vi "ir_laser_test.vi"() -> ()   [LabVIEW 2009]
uses:
  <vilib>/Utility/file.llb/Read From Spreadsheet File (string).vi
  <vilib>/Utility/error.llb/DialogType.ctl
  <vilib>/DAQmx/read.llb/DAQmx Read (Analog 2D DBL NChan NSamp).vi
  <vilib>/DAQmx/write.llb/DAQmx Write (Analog 1D DBL 1Chan NSamp).vi
  <vilib>/DAQmx/configure/timing.llb/DAQmx Timing (Sample Clock).vi
  <vilib>/DAQmx/create/channels.llb/DAQmx Create Channel (AO-Voltage-Basic).vi
  <vilib>/DAQmx/create/channels.llb/DAQmx Create Channel (AI-Voltage-Basic).vi
  <vilib>/Utility/file.llb/Write To Spreadsheet File (DBL).vi
  <vilib>/Analysis/NI_AALBase.lvlib
panel:
  in  "Start":bool
  in  "Exit":bool
  out "Selected pulse duration":dbl
  in  "Enable temp jump":bool
  in  "Select temperature jump":string(combo)
  in  "Cell name":string
  out "File overwritten":bool
  in  "Calculate Ea":bool
  out "standard error":string
  out "standard output":string
  in  "Activation energy":dbl=77000.0 caption="Activation energy [J/mol]" min=1000.0 max=2000000.0
  out "Estimated temperature":dbl[](graph)
  out "Laser control generated":dbl[](graph)
  in  "time between short pulses":dbl=1.0 caption="Time between short pulses [s]" format="%0.2p"
  in  "short pulse duration":dbl=1.0 caption="Short pulse duration [s]" format="%0.2p"
  in  "n short pulses":i32=3
  in  "Signal":u16(ring)=1 items=["Pulse train", "Simple pulse"]
  out "Current laser power [W]":dbl
  in  "Laser power [W]":dbl[](array[numeric]) min=0.0 max=10.0
  in  "repetitions":i32=3
  in  "Save file":bool=TRUE
  in  "filename":path
  out "Laser [W]":dbl[](graph) caption="Laser control"
  out "Temperature":dbl[](graph)
  out "Current [pA]":dbl[](graph) caption="Current"
  in  "Recording  duration":dbl=10.0 caption="Duration [s]" min=4.1 max=60.0 format="%0.2p"
  in  "Pulse duration":dbl=1.0 caption="Pulse duration [s]" min=0.001 max=1.5 format="%0.2p"
  in  "Amplitude":dbl=1.0 caption="Amplitude [W]" format="%0.2p"
  out "Measurement":dbl[][](graph)
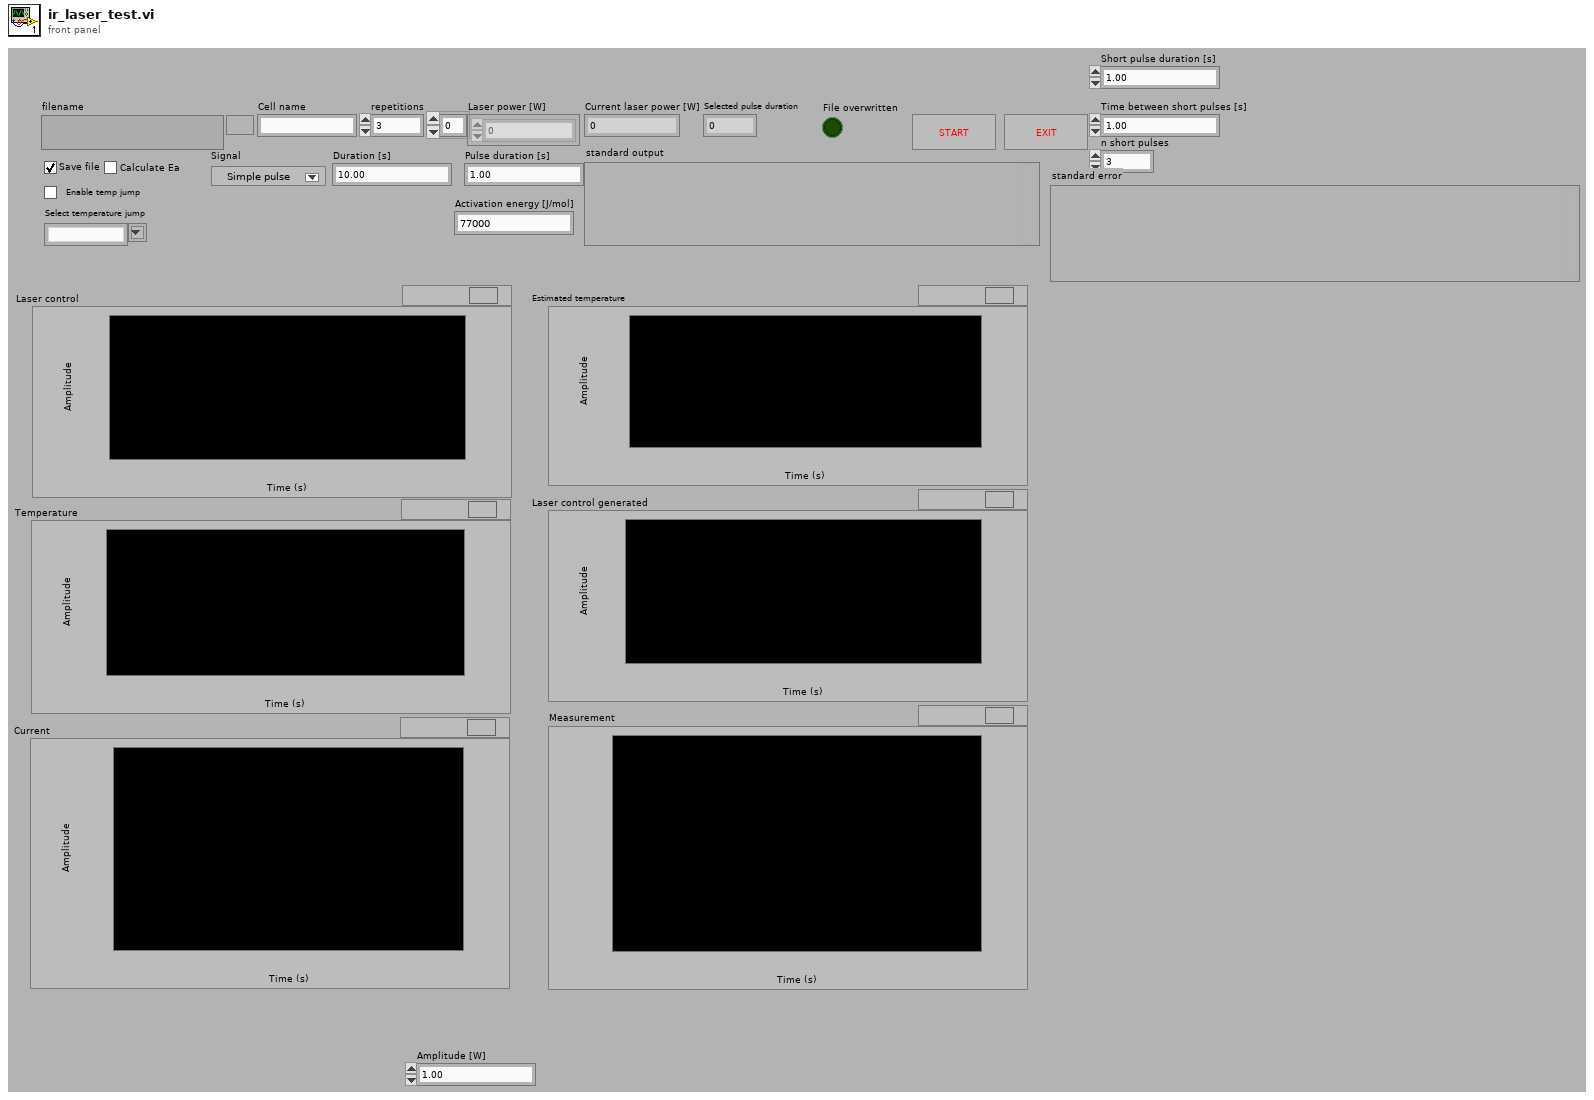
[diagram p1: front panel]
types:
  T1 = typedef "DialogType.ctl" = u16
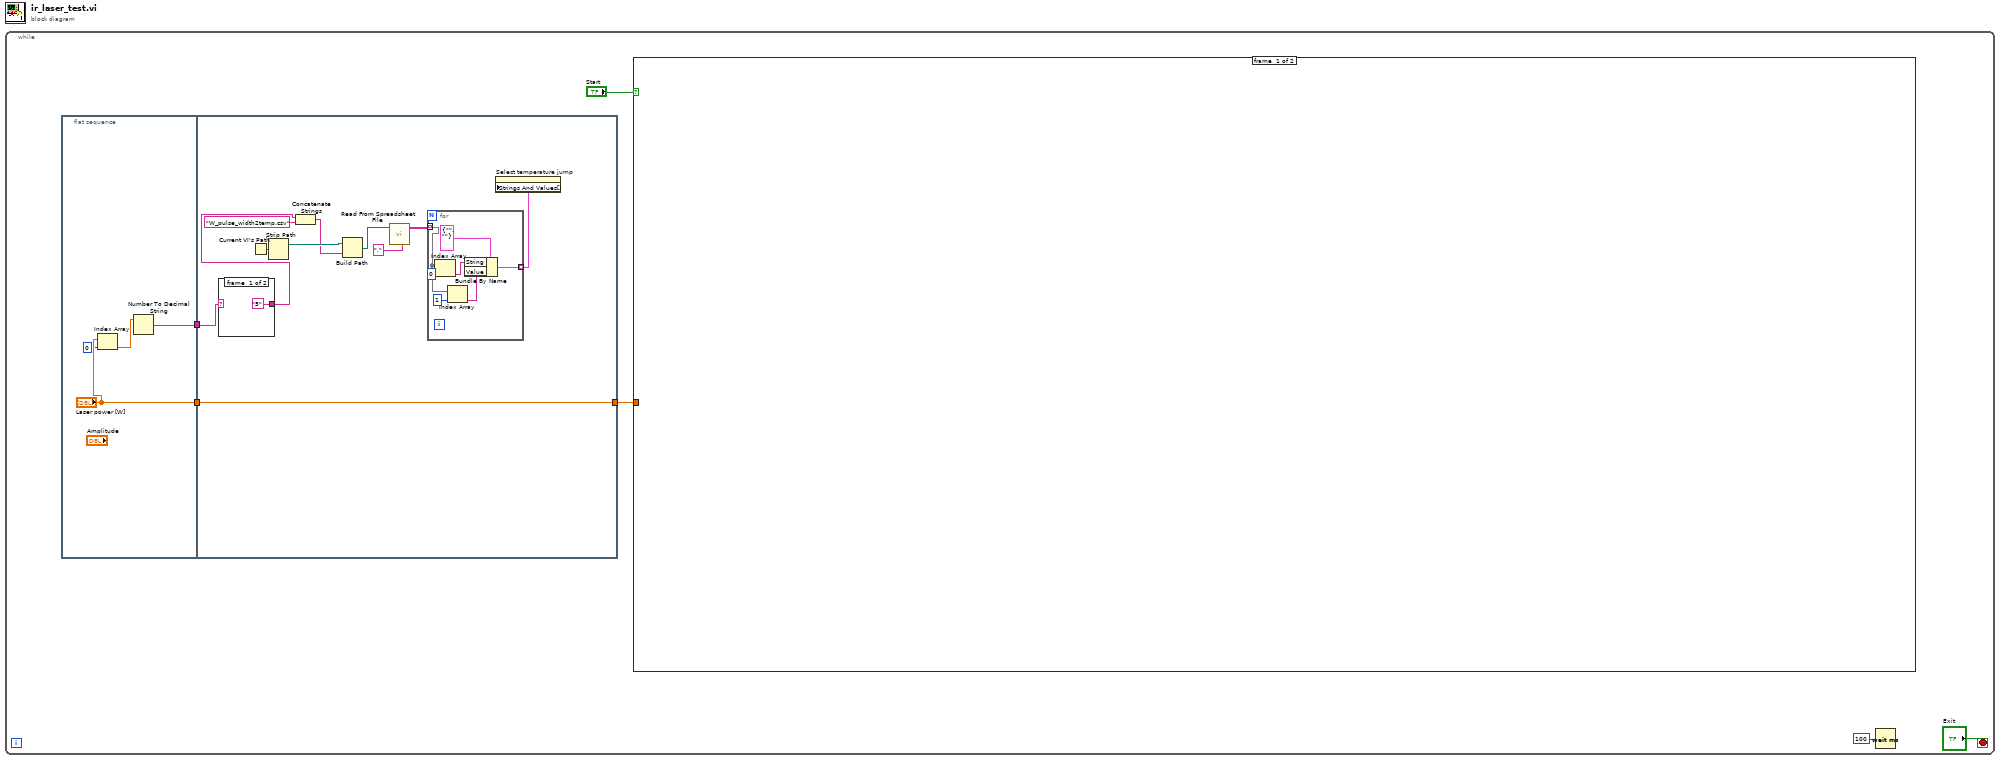
[diagram p0: block diagram]
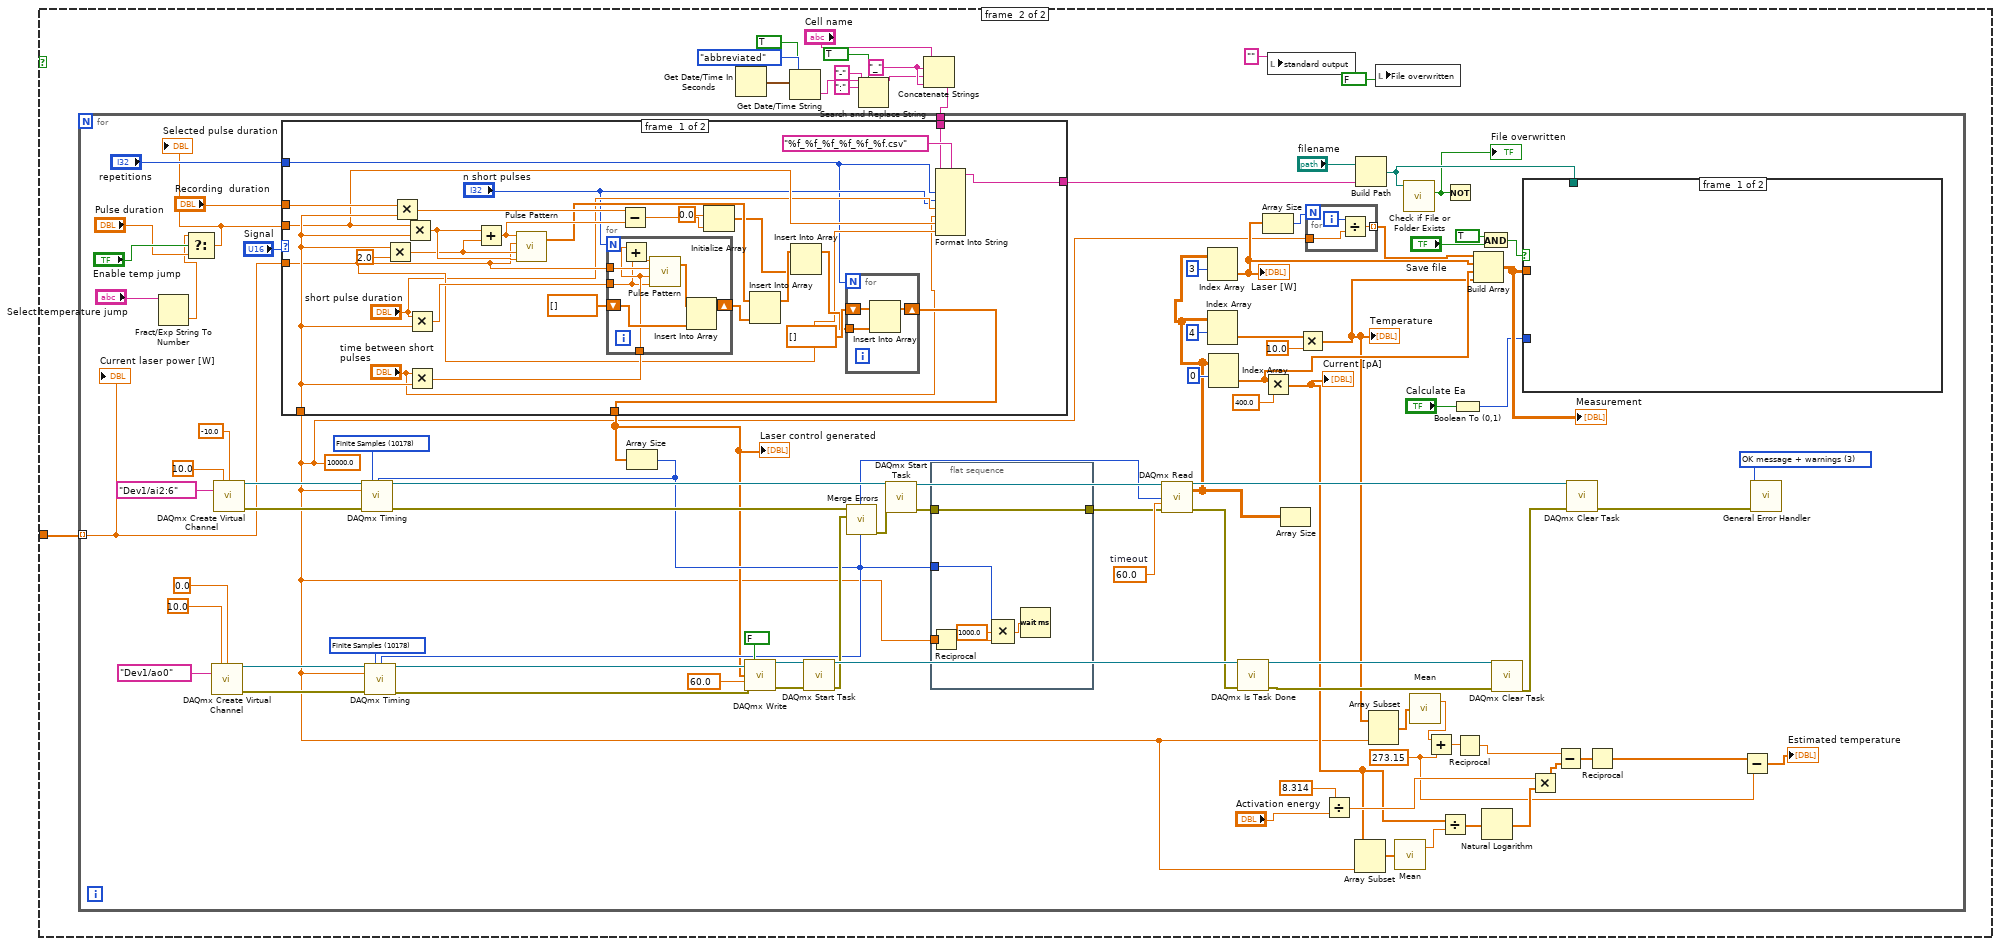
[diagram p2: hidden frame]
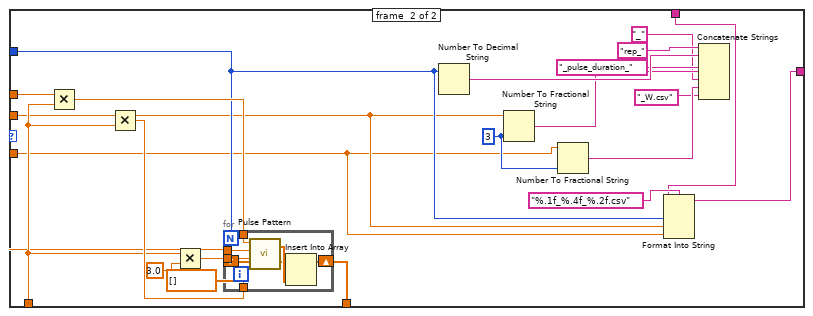
[diagram p3: hidden frame]
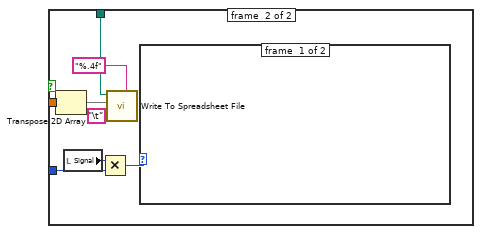
[diagram p4: hidden frame]
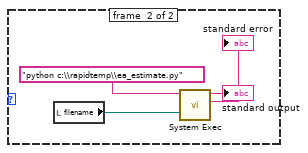
[diagram p5: hidden frame]
diagram:
  n1 = while {
    stop <- "Exit" stop-if-true
    n2 = flat-sequence {
      tunnel: ["Laser power [W]"] -> w6
      tunnel: [w195] -> w5
      tunnel: [w209] -> w4
      tunnel: w6 -> [w209]
      tunnel: w5 -> [w200]
      frame #0 {
        n3 = Index Array(array="Laser power [W]", index=0) -> (element=w196:dbl)
        n4 = Number To Decimal String(number=w196) -> (decimal integer string=w195:string)  [unwired: 1 in]
      }
      frame #1 {
        n5 = case shown="\"False\", Default" w200 {
          selector: w200 -> [_ w211]
          tunnel: ["5" w211] -> w199
          frame #0 {
          }
          frame #1 {
          }
        }
        n6 = Current VI's Path() -> (path=w206:path)
        n7 = Strip Path(path=w206) -> (stripped path=w208:path)  [unwired: 1 out]
        n8 = Concatenate Strings(w199, "W_pulse_width2temp.csv" ("string")) -> (w201:string)
        n9 = Build Path(base path=w208, name or relative path=w201) -> (appended path=w207:path)
        n10 = call-poly <vilib>:"Read From Spreadsheet File.vi"("delimiter (\\t)"="," ("delimiter (\\t)"), "file path (dialog if empty)"=w207) -> ("all rows"=w204:string[][])  [unwired: 5 in, 4 out]
        n11 = for {
          tunnel: w204 -> [w217] mode=indexing
          tunnel: [w212] -> w205 mode=indexing
          n12 = Index Array(array=w217, index=0) -> (element=w214:string)
          n13 = Index Array(array=w217, index=1) -> (element=w213:string)
          n14 = Bundle By Name(cluster=cluster{"String":string, "Value":string} {"String"="", "Value"=""} ("element"), "String"=w214, "Value"=w213) -> (w212:cluster{"String":string, "Value":string})
        }
        n15 = property on="Select temperature jump" class="CmbBox"("Strings And Values[]"=w205) -> ()  [unwired: 2 in, 2 out]
      }
    }
    n16 = case shown="True" "Start" {
      tunnel: w4 -> [_ w7]
      frame #0 {
      }
      frame #1 {
        w16 = "_" ("string")
        n17 = Get Date/Time In Seconds() -> (seconds since 1Jan1904=w15:timestamp)
        n18 = Get Date/Time String(date format (0)=enum16{"short", "long", "abbreviated"}."abbreviated", seconds (now)=w15, want seconds? (F)=TRUE) -> (time string=w11:string)  [unwired: 1 out]
        n19 = Search and Replace String(replace all?=TRUE ("replace all? (F)"), input string=w11, search string=":", replace string="-" ("replace string (\"\")")) -> (result string=w12:string)  [unwired: 4 in, 3 out]
        n20 = Concatenate Strings("Cell name", w16, w12, w16) -> (w17:string)
        n21 = for {
          tunnel: w7 -> [w56] mode=indexing
          tunnel: w17 -> [w30]
          w41 = 273.15 ("y")
          w82 = 60.0  # timeout
          w27 = 10000.0 ("Rate")
          w90 = T1 3 items=["no dialog", "OK message", "continue or stop message", "OK message + warnings", "continue/stop + warnings"] ("type of dialog (OK msg:1)")
          w97 = 10178 items=["Finite Samples"=10178, "Continuous Samples"=10123] ("sample mode")
          w103 = 10178 items=["Finite Samples"=10178, "Continuous Samples"=10123] ("sample mode")
          n22 = Fract/Exp String To Number(string="Select temperature jump") -> (number=w21:dbl)  [unwired: 3 in, 1 out]
          n23 = Select(t=w21, s="Enable temp jump", f="Pulse duration") -> (s? t:f=w23:dbl)
          "Selected pulse duration" <- w23
          n24 = call-poly <vilib>:"DAQmx Create Virtual Channel.vi"("maximum value"=10.0, "minimum value"=0.0, "physical channels"=tag "Dev1/ao0") -> ("task out"=w96:refnum<k21>, "error out"=w95:errorcluster)  [unwired: 11 in]
          n25 = call-poly <vilib>:"DAQmx Create Virtual Channel.vi"("maximum value"=10.0 ("Maximum Value"), "minimum value"=-10.0 ("Minimum Value"), "physical channels"=tag "Dev1/ai2:6" ("Physical Channel")) -> ("task out"=w101:refnum<k21>, "error out"=w102:errorcluster)  [unwired: 11 in]
          n26 = case shown="1" "Signal" {
            tunnel: "Recording  duration" -> [w137 w166]
            tunnel: "repetitions" -> [w111 w152]
            tunnel: w27 -> [w126 w163]
            tunnel: [w125 w149] -> w57
            tunnel: w23 -> [w121 w151]
            tunnel: w56 -> [w115 w150]
            tunnel: [w127 w154] -> w53
            tunnel: w30 -> [w110 w148]
            frame #0 {
              n27 = Multiply(x=w126, y=2.0) -> (x*y=w134:dbl)
              n28 = Multiply(x=w137, y=w126) -> (x*y=w133:dbl)
              n29 = Multiply(x=w121, y=w126) -> (x*y=w135:dbl)
              n30 = Multiply(x="short pulse duration", y=w126) -> (x*y=w123:dbl)
              n31 = Multiply(x="time between short pulses", y=w126) -> (x*y=w122:dbl)
              n32 = Add(x=w135, y=w134) -> (x+y=w132:dbl)
              n33 = call <vilib>:"Pulse Pattern.vi"("width"=w135, "delay"=w134, "amplitude"=w115, "samples"=w132) -> ("Pulse Pattern"=w129:dbl[])  [unwired: 1 out]
              n34 = for {
                N: "n short pulses" -> [_]
                tunnel: w115 -> [w144]
                tunnel: w123 -> [w141]
                shift-right: [w146] -> w130
                shift-left: dbl[] [] ("Pulse Pattern") -> [w145]
                tunnel: w122 -> [w142]
                n35 = Add(x=w142, y=w141) -> (x+y=w143:dbl)
                n36 = call <vilib>:"Pulse Pattern.vi"("width"=w141, "delay"=w142, "amplitude"=w144, "samples"=w143) -> ("Pulse Pattern"=w147:dbl[])  [unwired: 1 out]
                n37 = Insert Into Array(array=w147, new element=w145) -> (w146:dbl[])  [unwired: 1 in]
              }
              n38 = Subtract(x=w133, y=w132) -> (x-y=w120:dbl)
              n39 = Initialize Array(0.0 ("element"), w120) -> (w117:dbl[])
              n40 = Insert Into Array(array=w129, new element=w130) -> (w118:dbl[])  [unwired: 1 in]
              n41 = Insert Into Array(array=w118, new element=w117) -> (w116:dbl[])  [unwired: 1 in]
              n42 = for {
                N: w111 -> [_]
                tunnel: w116 -> [w140]
                shift-right: [w139] -> w127
                shift-left: dbl[] [] -> [w138]
                n43 = Insert Into Array(array=w138, new element=w140) -> (w139:dbl[])  [unwired: 1 in]
              }
              n44 = Format Into String(format string="%f_%f_%f_%f_%f_%f.csv", initial string=w110, w111, "n short pulses", "short pulse duration", "time between short pulses", w121, w115) -> (resulting string=w125:string)  [unwired: 1 in, 1 out]
            }
            frame #1 {
              w162 = i16 3 ("precision (6)")
              n45 = Multiply(x=w166, y=w163) -> (x*y=w165:dbl)
              n46 = Multiply(x=w151, y=w163) -> (x*y=w169:dbl)
              n47 = Multiply(x=w163, y=3.0) -> (x*y=w167:dbl)
              n48 = for {
                N: w152 -> [_]
                tunnel: w150 -> [w176]
                tunnel: w169 -> [w175]
                tunnel: w167 -> [w174]
                tunnel: w165 -> [w173]
                shift-right: [w172] -> w154
                shift-left: dbl[] [] -> [w170]
                n49 = call <vilib>:"Pulse Pattern.vi"("width"=w175, "delay"=w174, "amplitude"=w176, "samples"=w173) -> ("Pulse Pattern"=w171:dbl[])  [unwired: 1 out]
                n50 = Insert Into Array(array=w170, new element=w171) -> (w172:dbl[])  [unwired: 1 in]
              }
              n51 = Number To Decimal String(number=w152) -> (decimal integer string=w160:string)  [unwired: 1 in]
              n52 = Number To Fractional String(number=w151, precision (6)=w162) -> (F-format string=w158:string)  [unwired: 2 in]
              n53 = Number To Fractional String(number=w150, precision (6)=w162) -> (F-format string=w156:string)  [unwired: 2 in]
              n54 = Format Into String(format string="%.1f_%.4f_%.2f.csv", initial string=w148, w152, w151, w150) -> (resulting string=w149:string)  [unwired: 1 in, 1 out]
              n55 = Concatenate Strings("rep_" ("string"), w160, "_pulse_duration_" ("string"), w158, "_" ("string"), w156, "_W.csv" ("format string")) -> ()  [unwired: 1 out]
            }
          }
          "Laser control generated" <- w53
          n56 = Array Size(array=w53) -> (size(s)=w54:i32)
          n57 = call-poly <vilib>:"DAQmx Timing.vi"("task/channels in"=w101, "sample mode"=w103, "samples per channel"=w54, "rate"=w27, "error in"=w102) -> ("task out"=w67:refnum<k21>, "error out"=w68:errorcluster)  [unwired: 9 in]
          n58 = call-poly <vilib>:"DAQmx Timing.vi"("task/channels in"=w96, "sample mode"=w97, "samples per channel"=w54, "rate"=w27, "error in"=w95) -> ("task out"=w65:refnum<k21>, "error out"=w66:errorcluster)  [unwired: 9 in]
          n59 = call-poly <vilib>:"DAQmx Write.vi"("task/channels in"=w65, "auto start"=FALSE, "data"=w53, "timeout"=60.0 ("Wirite Timeout"), "error in"=w66) -> ("task out"=w92:refnum<k21>, "error out"=w91:errorcluster)  [unwired: 8 in, 1 out]
          n60 = call <vilib>:"DAQmx Start Task.vi"("task/channels in"=w92, "error in"=w91) -> ("task out"=w94:refnum<k21>, "error out"=w87:errorcluster)  [unwired: 12 in]
          n61 = call <vilib>:"Merge Errors.vi"("error in 2 (no error)"=w87, "error in 1 (no error)"=w68) -> ("error out"=w86:errorcluster)  [unwired: 5 in]
          n62 = call <vilib>:"DAQmx Start Task.vi"("task/channels in"=w67, "error in"=w86) -> ("task out"=w88:refnum<k21>, "error out"=w72:errorcluster)  [unwired: 12 in]
          n63 = flat-sequence {
            tunnel: w72 -> [w194]
            tunnel: [w194] -> w71
            tunnel: w54 -> [w193]
            tunnel: w27 -> [w190]
            frame #0 {
              n64 = Reciprocal(x=w190) -> (1/x=w189:dbl)
              n65 = Compound Arithmetic op=MULTIPLY(w193, 1000.0 ("y"), w189) -> (w192:dbl)
              n66 = Wait (ms)(milliseconds to wait=w192) -> ()  [unwired: 1 out]
            }
          }
          n67 = call-poly <vilib>:"DAQmx Read.vi"("task/channels in"=w88, "number of samples per channel"=w54, "timeout"=w82, "error in"=w71) -> ("task out"=w104:refnum<k21>, "data"=w75:dbl[][], "error out"=w81:errorcluster)  [unwired: 9 in]
          n68 = Index Array(array=w75, index (row)=3) -> (element=w29:dbl[])  [unwired: 1 in]
          "Laser [W]" <- w29
          n69 = Index Array(array=w75, index (row)=4) -> (element=w79:dbl[])  [unwired: 1 in]
          n70 = Index Array(array=w75, index (row)=0) -> (element=w61:dbl[])  [unwired: 1 in]
          n71 = call <vilib>:"DAQmx Is Task Done.vi"("task/channels in"=w94, "error in"=w81) -> ("task out"=w93:refnum<k21>, "error out"=w85:errorcluster)  [unwired: 11 in, 1 out]
          n72 = Array Size(array=w29) -> (size(s)=w28:i32)
          n73 = Multiply(x=w61, y=400.0 ("Minimum Value")) -> (x*y=w35:dbl[])
          "Current [pA]" <- w35
          n74 = Array Size(array=w75) -> ()  [unwired: 1 out]
          n75 = Multiply(x=w79, y=10.0 ("Minimum Value")) -> (x*y=w40:dbl[])
          "Temperature" <- w40
          n76 = for {
            N: w28 -> [_]
            tunnel: w27 -> [w108]
            tunnel: [w107] -> w26 mode=indexing
            i -> [w109]
            n77 = Divide(x=w109, y=w108) -> (x/y=w107:dbl)
          }
          n78 = Divide(x=8.314, y="Activation energy") -> (x/y=w49:dbl)
          n79 = Array Subset(array=w35, length=w27) -> (w36:dbl[])  [unwired: 1 in]
          n80 = Build Path(base path="filename", name or relative path=w57) -> (appended path=w59:path)
          n81 = Array Subset(array=w40, length=w27) -> (w39:dbl[])  [unwired: 1 in]
          n82 = call <vilib>:"Mean.vi"("X"=w36) -> ("mean"=w37:dbl)  [unwired: 1 out]
          n83 = call <vilib>:"Check if File or Folder Exists.vi"("path"=w59) -> ("file or folder exists?"=w31:bool)  [unwired: 8 in, 2 out]
          "File overwritten" <- w31
          n84 = call <vilib>:"Mean.vi"("X"=w39) -> ("mean"=w38:dbl)  [unwired: 1 out]
          n85 = Add(x=w38, y=w41) -> (x+y=w52:dbl)
          n86 = Divide(x=w35, y=w37) -> (x/y=w50:dbl[])
          n87 = Not(x=w31) -> ()  [unwired: 1 out]
          n88 = Boolean To (0,1)(Boolean="Calculate Ea") -> (0, 1=w32:i16)
          n89 = Reciprocal(x=w52) -> (1/x=w44:dbl)
          n90 = Build Array(w26, w29, w61, w40) -> (w63:dbl[][])
          "Measurement" <- w63
          n91 = And(x=TRUE, y="Save file") -> (x .and. y?=w62:bool)
          n92 = Natural Logarithm(1:w50) -> (0:w46:dbl[])
          n93 = call <vilib>:"DAQmx Clear Task.vi"("task in"=w93, "error in"=w85) -> ("error out"=w84:errorcluster)  [unwired: 13 in]
          n94 = case shown="True" w62 {
            tunnel: w63 -> [_ w184]
            tunnel: w59 -> [_ w182]
            tunnel: w32 -> [_ w179]
            frame #0 {
            }
            frame #1 {
              n95 = Transpose 2D Array(2D array=w184) -> (transposed array=w178:dbl[][])
              n96 = local read "Signal"() -> (w181:u16)
              n97 = Multiply(x=w181, y=w179) -> (x*y=w180:u16)
              n98 = call-poly <vilib>:"Write To Spreadsheet File.vi"("delimiter (\\t)"="\t" ("delimiter (\\t)"), "format (%.3f)"="%.4f", "2D data"=w178, "file path (dialog if empty)"=w182) -> ()  [unwired: 4 in, 1 out]
              n99 = case shown="1" w180 {
                frame #0 {
                }
                frame #1 {
                  n100 = local read "filename"() -> (w186:path)
                  n101 = call <vilib>:"System Exec.vi"("working directory"=w186, "command line"="python c:\\rapidtemp\\ea_estimate.py") -> ("standard error"=→"standard error":string, "standard output"=→"standard output":string)  [unwired: 6 in, 2 out]
                }
              }
            }
          }
          n102 = Multiply(x=w49, y=w46) -> (x*y=w47:dbl[])
          n103 = Subtract(x=w44, y=w47) -> (x-y=w48:dbl[])
          n104 = call <vilib>:"DAQmx Clear Task.vi"("task in"=w104, "error in"=w84) -> ("error out"=w83:errorcluster)  [unwired: 13 in]
          n105 = Reciprocal(x=w48) -> (1/x=w42:dbl[])
          n106 = Subtract(x=w42, y=w41) -> (x-y=→"Estimated temperature":dbl[])
          n107 = call <vilib>:"General Error Handler.vi"("type of dialog (OK msg:1)"=w90, "error in (no error)"=w83) -> ()  [unwired: 9 in, 5 out]
          "Current laser power [W]" <- w56
        }
        n108 = local write "standard output"("" ("standard output")) -> ()
        n109 = local write "File overwritten"(FALSE ("File overwritten")) -> ()
      }
    }
    n110 = Wait (ms)(milliseconds to wait=u32 100) -> ()  [unwired: 1 out]
  }
